vi "post step shake.vi"(8 "error in (no error)":errorcluster, 11 "TapeDrive in":refnum<class "TapeDrive.lvclass">) -> (0 "error out":errorcluster, 3 "TapeDrive out":refnum<class "TapeDrive.lvclass">)   [LabVIEW 2020, in "TapeDrive.lvclass"]
uses:
  TapeDrive.lvclass
  TapeDrive.lvclass/TapeDrive.ctl
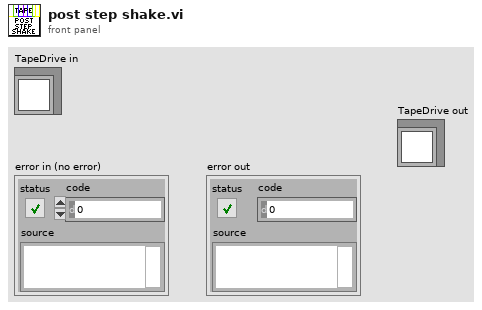
[diagram p1: front panel]
types:
  T1 = typedef "OnOffTypeDef.ctl" = enum16{"off", "on"}
  T2 = typedef "Direction_TypDef.ctl" = enum16{"left", "right"}
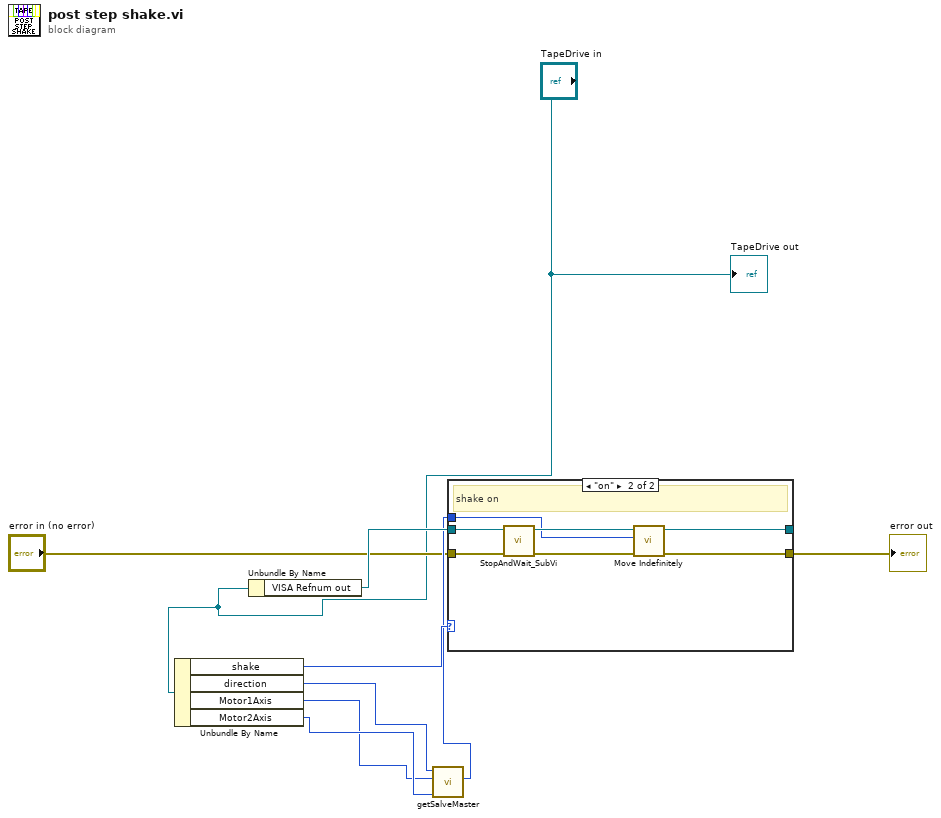
[diagram p0: block diagram]
diagram:
  n1 = Unbundle By Name("TapeDrive in") -> ("shake"=w8:T1, "direction"=w4:T2, "Motor1Axis"=w5:i32, "Motor2Axis"=w6:i32)
  n2 = Unbundle By Name("TapeDrive in") -> ("VISA Refnum out"=w9:refnum<visa-resource-name>)
  n3 = call "getSalveMaster.vi"("Motor2Axis"=w6, "Motor1Axis"=w5, "direction"=w4) -> ("Master"=w7:i32)  [unwired: 7 in, 1 out]
  n4 = case shown="\"on\"" w8 {
    tunnel: w9 -> [w11 w18]
    tunnel: [w11 w16] -> _
    tunnel: w7 -> [_ w15]
    tunnel: "error in (no error)" -> [w10 w14]
    tunnel: [w10 w12] -> w2
    frame "off", Default {
    }
    frame "on" {
      # "shake on"
      n5 = call "StopAndWait_SubVi.vi"("error in (no error)"=w14, "VISA Refnum in"=w18) -> ("error out"=w13:errorcluster, "VISA Refnum out"=w17:refnum<visa-resource-name>)  [unwired: 8 in]
      n6 = call "Move Indefinitely.vi"("error in (no error)"=w13, "Axis (1)"=w15, "VISA resource name"=w17) -> ("error out"=w12:errorcluster, "VISA resource name out"=w16:refnum<visa-resource-name>)  [unwired: 3 in]
    }
  }
  "error out" <- w2
  "TapeDrive out" <- "TapeDrive in"
